vi "init_hw.vi"(8 "error in (no error)":errorcluster, 11 "ibsen in":refnum<class "ibsen.lvclass">) -> (0 "error out":errorcluster, 2 "success ?":bool=TRUE, 3 "ibsen out":refnum<class "ibsen.lvclass">)   [LabVIEW 2019, in "ibsen.lvlib" / "ibsen.lvclass"]
uses:
  ibsen.lvclass
  D:/github/TransientAbsorptionDAQ.lv/_camera/_camera.lvlibp/_cameraClass/_camera.lvclass
  ibsen.lvclass/ibsen.ctl
  _camera/_camera.lvlibp/_cameraClass/Write wavelength.vi
panel:
  out "size(s)":i32
  out "Array":dbl[](array[numeric])
  out "concatenated string":string
  # "Loading hardware ..."
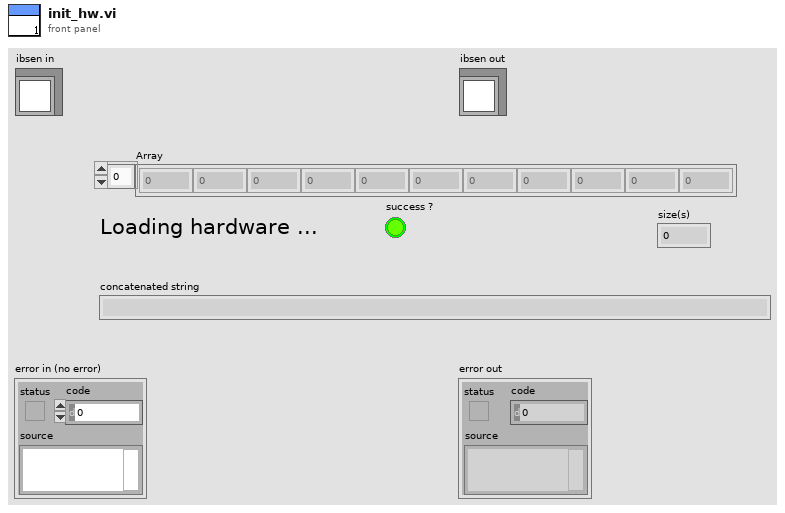
[diagram p1: front panel]
types:
  T1 = cluster{"Read Access":enum8{"Allowed", "Required", "None"}, "Write Access":enum8{"Allowed", "Required", "None"}}
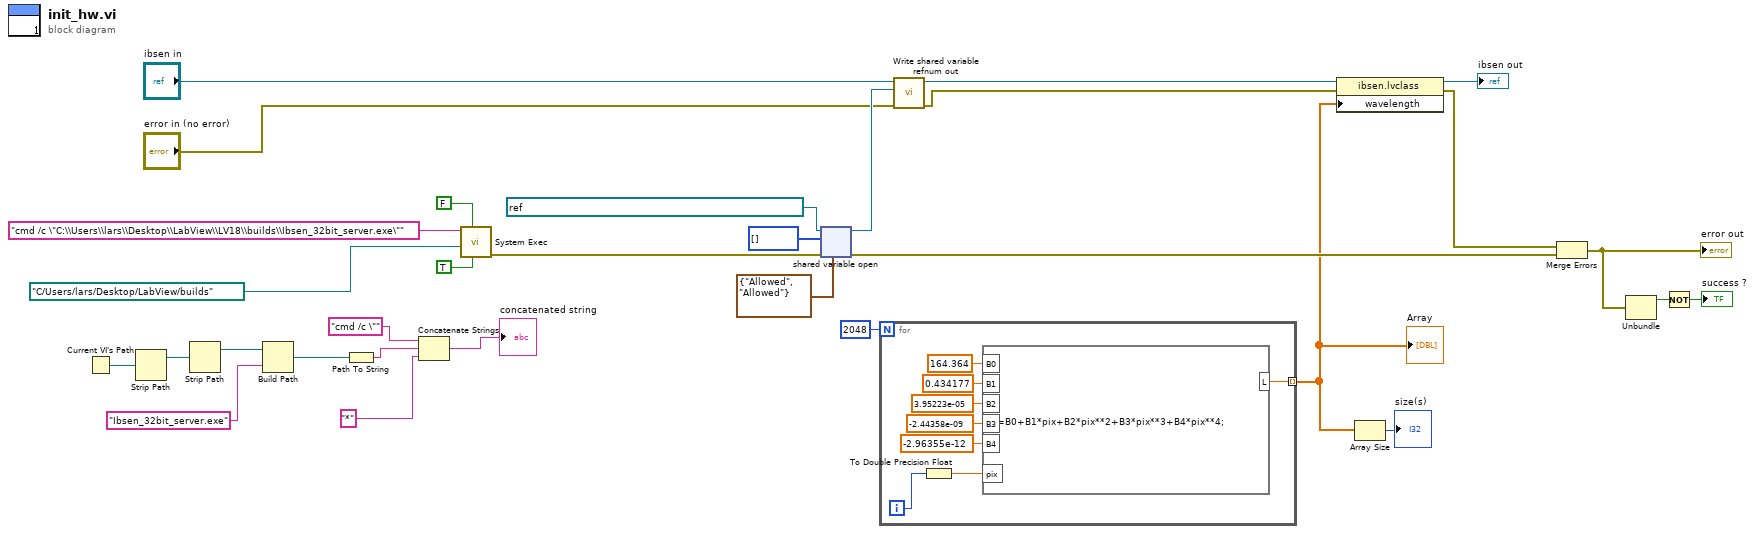
[diagram p0: block diagram]
diagram:
  n1 = Current VI's Path() -> (path=w21:path)
  n2 = Strip Path(path=w21) -> (stripped path=w20:path)  [unwired: 1 out]
  n3 = Strip Path(path=w20) -> (stripped path=w19:path)  [unwired: 1 out]
  n4 = Build Path(base path=w19, name or relative path="Ibsen_32bit_server.exe") -> (appended path=w17:path)
  n5 = Path To String(path=w17) -> (string=w15:string)
  n6 = Concatenate Strings("cmd /c \"", w15, "*") -> (→"concatenated string":string)
  n7 = call <vilib>:"System Exec.vi"("run minimized? (F)"=TRUE, "wait until completion? (T)"=FALSE, "working directory"=path "C:/Users/lars/Desktop/LabView/builds", "command line"="cmd /c \"C:\\Users\\lars\\Desktop\\LabView\\LV18\\builds\\Ibsen_32bit_server.exe\"") -> ("error out"=w27:errorcluster)  [unwired: 4 in, 3 out]
  n8 = shared-variable-open(refnum<k21> "ni.var.psp://localhost/Ibsen_background/spectrum" ("shared variable refnum in"), w27, i32[] [], T1 {"Read Access"=enum."Allowed", "Write Access"=enum."Allowed"} ("access")) -> (w28:refnum<k21>, w11:errorcluster)
  n9 = for {
    N: 2048 -> [_]
    tunnel: [w33] -> w2 mode=indexing
    i -> [w34]
    n10 = To Double Precision Float(number=w34) -> (double precision float=w32:dbl)
    n11 = formula code="L=B0+B1*pix+B2*pix**2+B3*pix**3+B4*pix**4;"("B0"=164.364, "B1"=0.434177 ("input variable"), "B2"=3.95223e-05 ("input variable"), "B3"=-2.44358e-09 ("input variable"), "B4"=-2.96355e-12 ("input variable"), "pix"=w32) -> ("L"=w33:dbl)
  }
  "Array" <- w2
  n12 = call "Write shared variable refnum out.vi"("error in (no error)"="error in (no error)", "shared variable refnum out"=w28, "ibsen in"="ibsen in") -> ("error out"=w5:errorcluster, "ibsen out"=w7:refnum<class "ibsen.lvclass">)  [unwired: 7 in]
  n13 = property class="ibsen.lvclass"(reference=w7, error in=w5, "wavelength"=w2) -> (reference out=→"ibsen out":refnum<class "ibsen.lvclass">, error out=w4:errorcluster)
  n14 = Array Size(array=w2) -> (size(s)=→"size(s)":i32)
  n15 = Merge Errors(w4, w11) -> (w10:errorcluster)
  "error out" <- w10
  n16 = Unbundle(w10) -> ("status"=w8:bool)  [unwired: 2 out]
  n17 = Not(x=w8) -> (.not. x?=→"success ?":bool)
